vi "Write Client Count.vi"(10 "Client Count":i32, 11 "Client in":refnum<class "Client.lvclass">) -> (3 "Client out":refnum<class "Client.lvclass">)   [LabVIEW 2016, in "Client.lvlib" / "Client.lvclass"]
uses:
  Client.lvclass
  Client.lvclass/Client.ctl
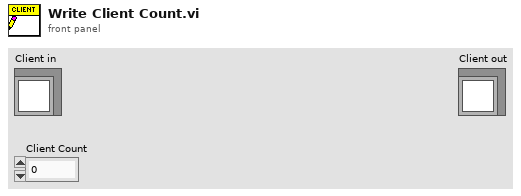
[diagram p1: front panel]
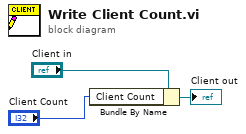
[diagram p0: block diagram]
diagram:
  n1 = Bundle By Name(cluster="Client in", "Client Count"="Client Count") -> (→"Client out":refnum<class "Client.lvclass">)
